vi "Generate Profile.vi"() -> ()   [LabVIEW 2019]
uses:
  Motion Profile Generator/Type Defs/Control Boundaries.ctl
  Motion Profile Generator/Type Defs/Motion Snapshot.ctl
  Motion Profile Generator/Motion Profile Generator.lvclass/Motion Profile Generator.ctl
  Motion Profile Generator/Public Methods/Read Motion Profile Array.vi
  Motion Profile Generator/Motion Profile Generator.lvclass
panel:
  in  "Create file?":bool
  in  "Distance (in)":dbl=50.0 format="%#_13g"
  in  "Starting Conditions":T1
  in  "Control Boundaries":T2={"Max Speed (in/s)"=5.0, "Max Acceleration (in/s2)"=3.0, "Max Deceleration (in/s2)"=0.0}
  out "Steps":i32
  out "Duration (s)":dbl
  out "XY Graph":cluster{dbl[], dbl[]}[](graph)
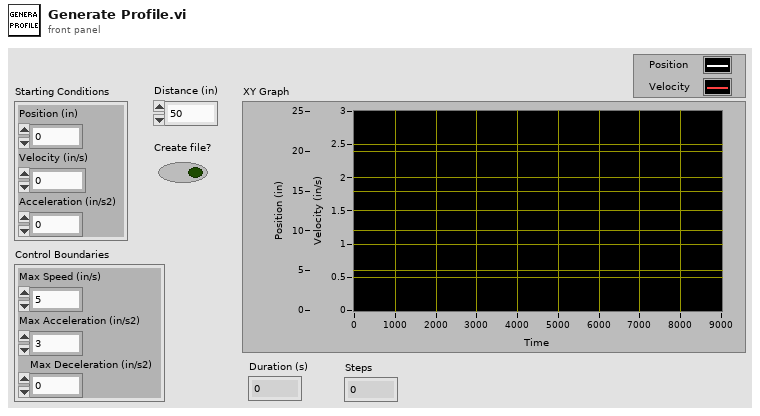
[diagram p1: front panel]
types:
  T1 = typedef "Motion Profile Generator.lvclass/Motion Snapshot.ctl" = cluster{"Position (in)":dbl, "Velocity (in/s)":dbl, "Acceleration (in/s2)":dbl}
  T2 = typedef "Motion Profile Generator.lvclass/Control Boundaries.ctl" = cluster{"Max Speed (in/s)":dbl, "Max Acceleration (in/s2)":dbl, "Max Deceleration (in/s2)":dbl}
  T3 = typedef "Motion Profile Generator.lvclass/Motion Profile Point.ctl" = cluster{"Position (in)":dbl, "Velocity (in/s)":dbl, "Duration (ms)":dbl}
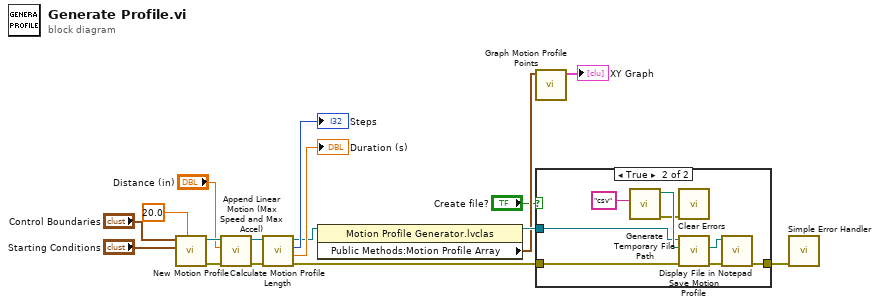
[diagram p0: block diagram]
diagram:
  n1 = call "New Motion Profile.vi"("Time Between Points (ms)"=20.0, "Starting Conditions"="Starting Conditions", "Control Boundaries"="Control Boundaries") -> ("error out"=w17:errorcluster, "Motion Profile Generator out"=w11:refnum<class "Motion Profile Generator.lvclass">)  [unwired: 7 in]
  n2 = call "Append Linear Motion (Max Speed and Max Accel).vi"("error in (no error)"=w17, "Distance (in)"="Distance (in)", "Motion Profile Generator in"=w11) -> ("error out"=w12:errorcluster, "Motion Profile Generator out"=w9:refnum<class "Motion Profile Generator.lvclass">)  [unwired: 7 in]
  n3 = call "Calculate Motion Profile Length.vi"("error in (no error)"=w12, "Motion Profile Generator in"=w9) -> ("error out"=w1:errorcluster, "Duration (s)"=→"Duration (s)":dbl, "Steps"=→"Steps":i32, "Motion Profile Generator out"=w6:refnum<class "Motion Profile Generator.lvclass">)  [unwired: 5 in, 1 out]
  n4 = property class="Motion Profile Generator.lvclas"(reference=w6) -> (reference out=w5:refnum<class "Motion Profile Generator.lvclass">, "Public Methods:Motion Profile Array"=w4:T3[])  [unwired: 1 in, 1 out]
  n5 = call "Graph Motion Profile Points.vi"("Motion Profile Array"=w4) -> ("Array"=→"XY Graph":cluster{dbl[], dbl[]}[])  [unwired: 10 in]
  n6 = case shown="True" "Create file?" {
    tunnel: [w18 w21] -> w16
    tunnel: w1 -> [w18 w20]
    tunnel: w5 -> [_ w19]
    frame False {
    }
    frame True {
      n7 = call <vilib>:"Generate Temporary File Path.vi"("Temporary File Extension (tmp)"="csv") -> ("error out"=w24:errorcluster, "Unique Temporary File Path"=w25:path)  [unwired: 9 in]
      n8 = call <vilib>:"Clear Errors.vi"("error in (no error)"=w24) -> ()  [unwired: 5 in, 2 out]
      n9 = call "Save Motion Profile.vi"("error in (no error)"=w20, "File Path (.csv)"=w25, "Motion Profile Generator in"=w19) -> ("error out"=w22:errorcluster, "New File Path (.csv)"=w23:path)  [unwired: 6 in, 1 out]
      n10 = call "Display File in Notepad.vi"("error in"=w22, "File Path"=w23) -> ("error out"=w21:errorcluster)  [unwired: 9 in]
    }
  }
  n11 = call <vilib>:"Simple Error Handler.vi"("error in (no error)"=w16) -> ()  [unwired: 4 in, 5 out]
